vi "Main.vi"() -> ()   [LabVIEW 2021]
doc: "This template is for the Queued Message Handler design pattern.\n\nThe Event Handling Loop generates messages based on user interface actions.\n\nThe Message Handling Loop processes messages generated by the Event Handling Loop, or by other messages. The messages are string values, so new messages can be added easily to the Message Cases case structure in the Message Handling Loop. Each message cluster can also provide an optional value for Message Data, which is a variant that can be converted to whatever message-specific data is required."
uses:
  Controls/Status Lights.ctl
  controls/UI Data.ctl
  support/Message Queue/Enqueue Message (Single).vi
  <vilib>/Utility/error.llb/Error Cluster From Error Code.vi
  <vilib>/ErrorRing/Error Ring.xnode
  support/Message Queue/Message Queue.lvlib
  support/User Event - Stop/User Event - Stop.lvlib
panel:
  out "Status":T1
  in  "Speed":dbl(knob) scale=0.0..10.0
  out "Display":string
  in  "Direction":bool
  in  "Apply Brake":bool
  in  "Exit":bool
  # "These controls have associated \"Value Changed\" events configured in the Event Structure on the diagram.\n\nReplace them (and reconfigure the Event Structure) with the controls you need for your application."
  # "This template is for the Queued Message Handler design pattern.\n\nSee the block diagram for more information on how to use this template."
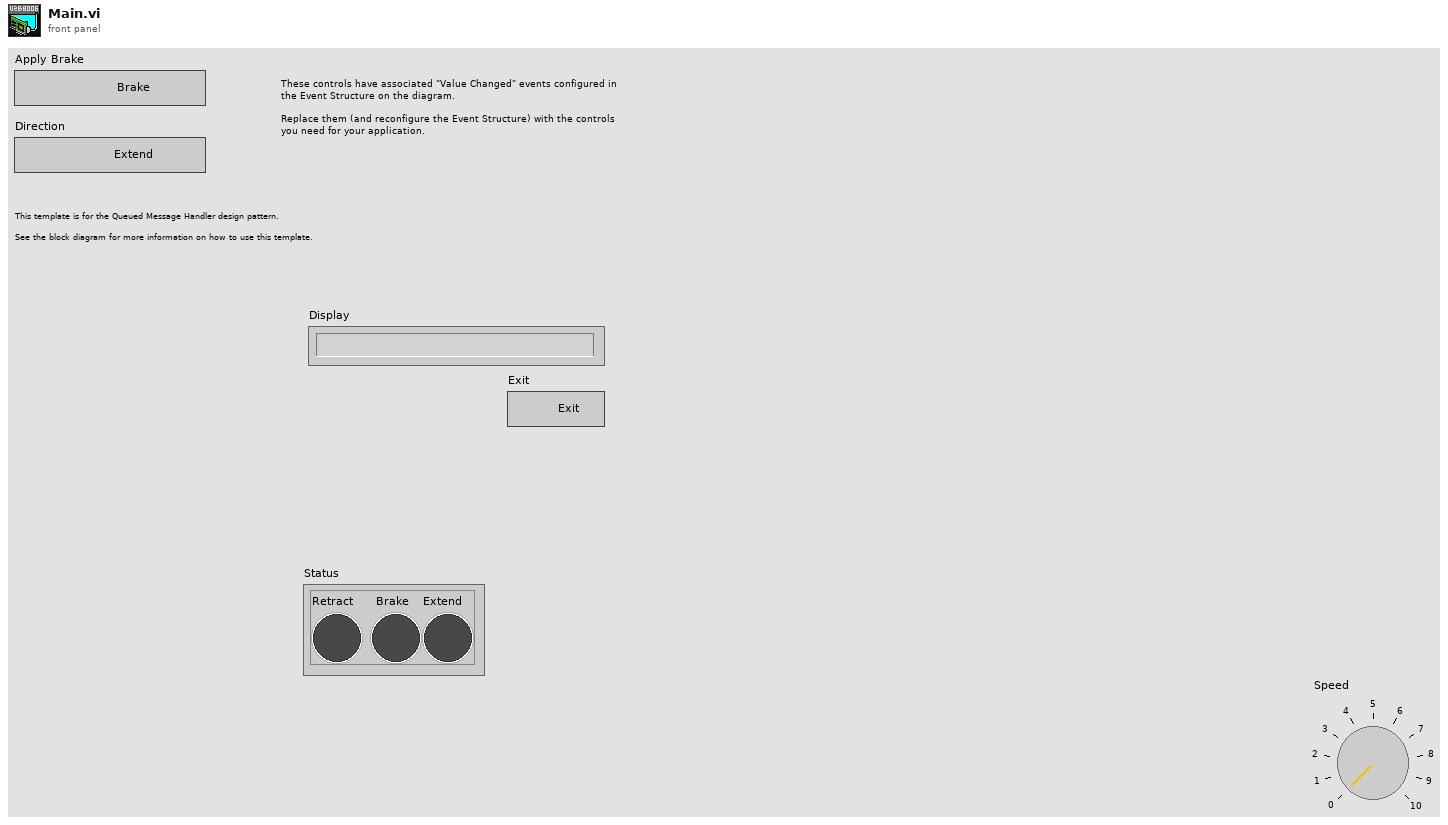
[diagram p1: front panel]
types:
  T1 = typedef "Status Lights.ctl" = cluster{"Retract":bool, "Brake":bool, "Extend":bool}
  T2 = typedef "UI Data.ctl" = cluster{"Boolean":bool, "String":string, "Velocity":dbl, "Apply Brake Ref":refnum<vi>, "Direction Ref":refnum<vi>, "Data Display Ref":refnum<vi>, "Exit Button Ref":refnum<vi>, "Status":T1}
  T3 = typedef "Message Queue.lvlib/All Message Queues.ctl" = cluster{"UI":refnum<queue>}
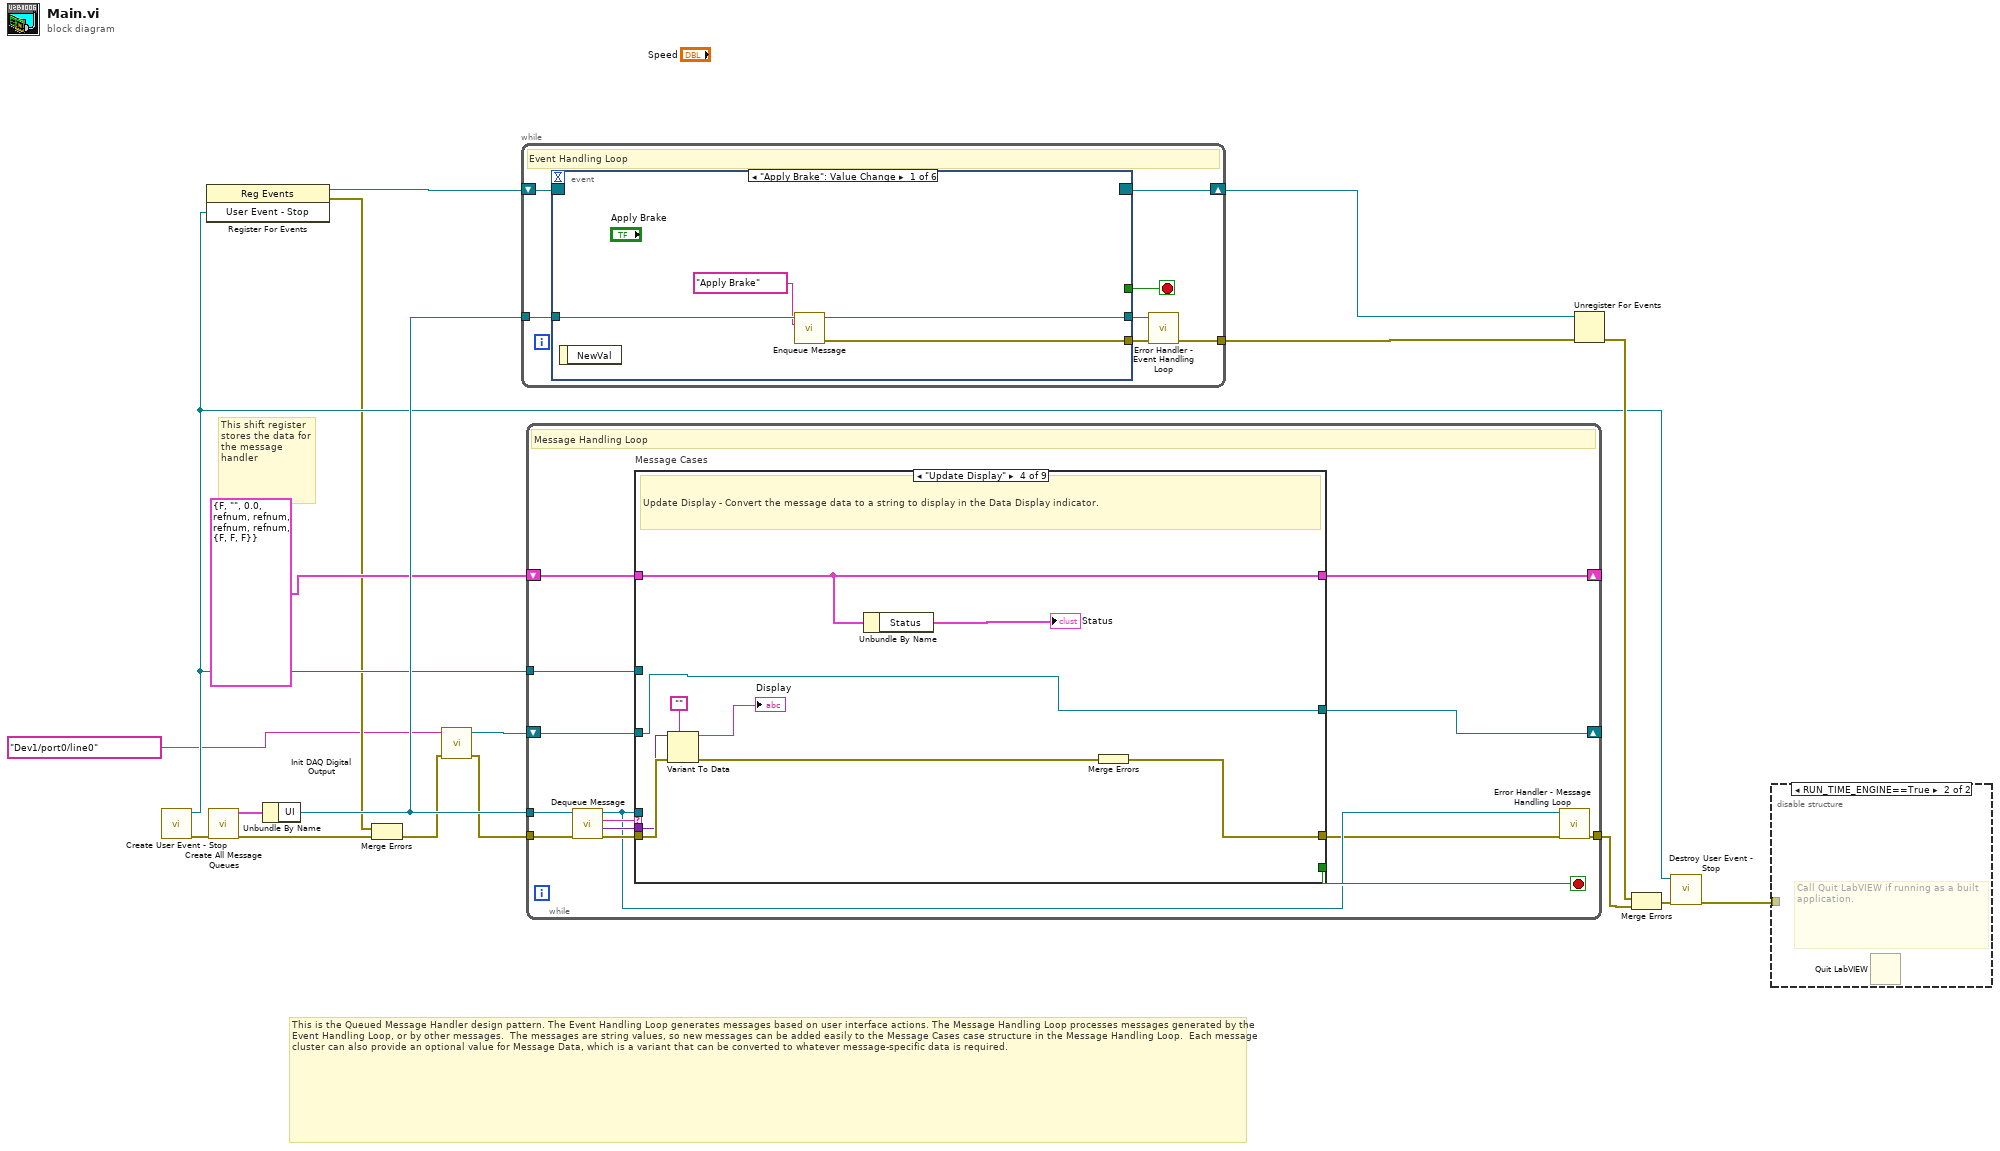
[diagram p0: block diagram]
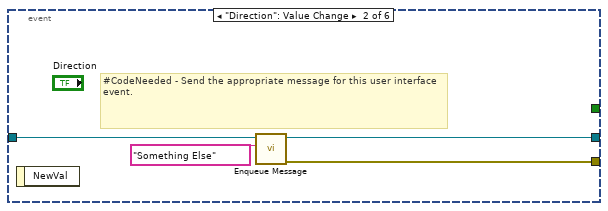
[diagram p3: hidden frame]
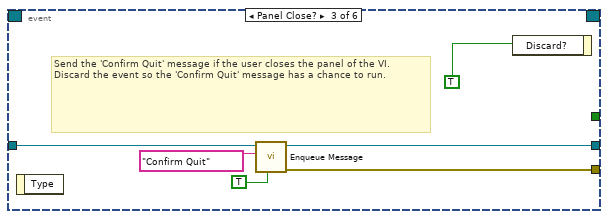
[diagram p4: hidden frame]
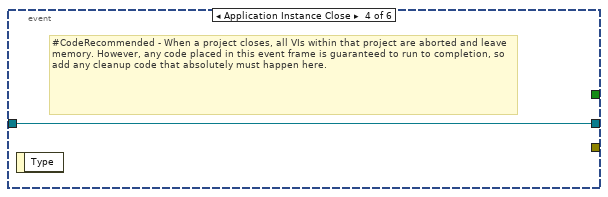
[diagram p5: hidden frame]
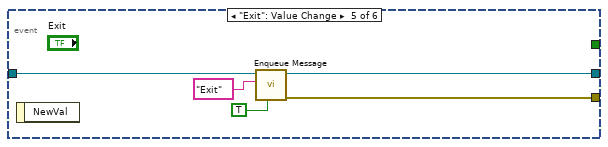
[diagram p6: hidden frame]
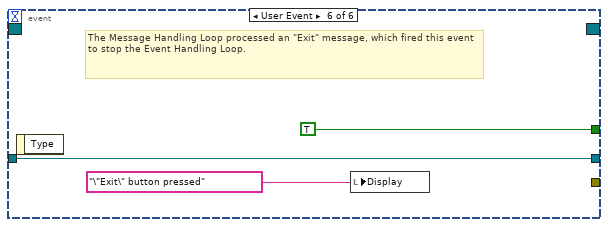
[diagram p7: hidden frame]
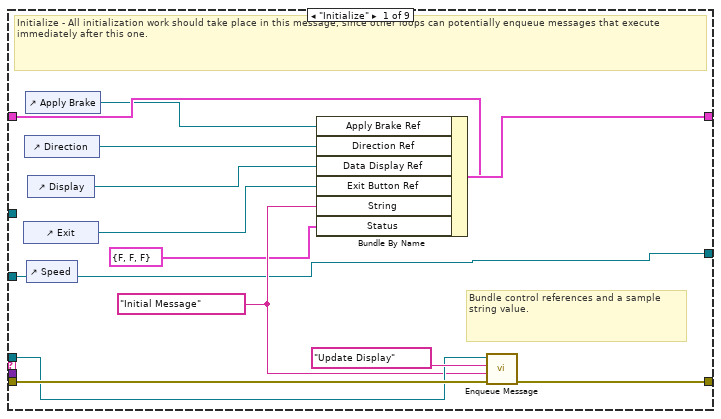
[diagram p8: hidden frame]
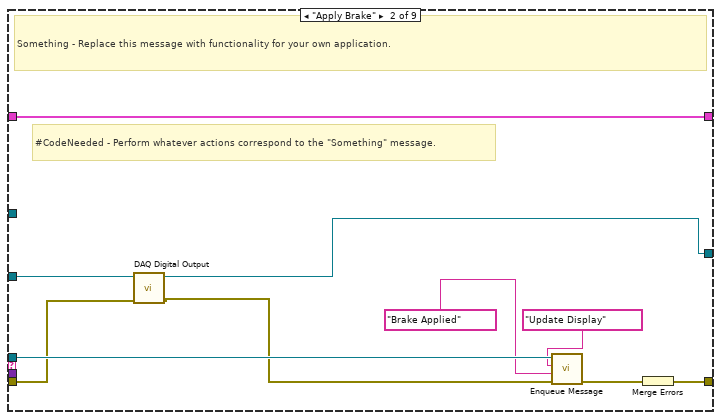
[diagram p9: hidden frame]
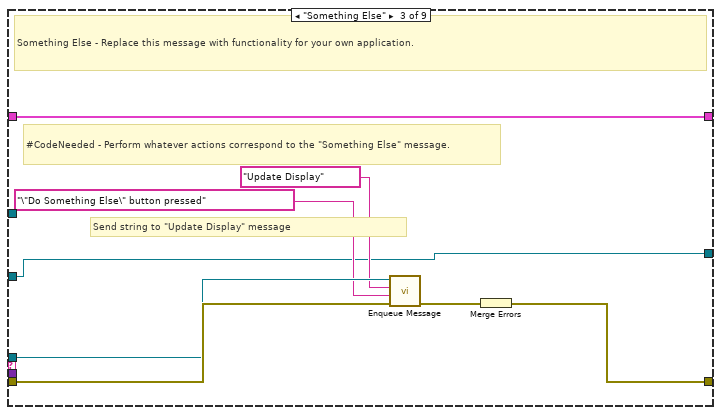
[diagram p10: hidden frame]
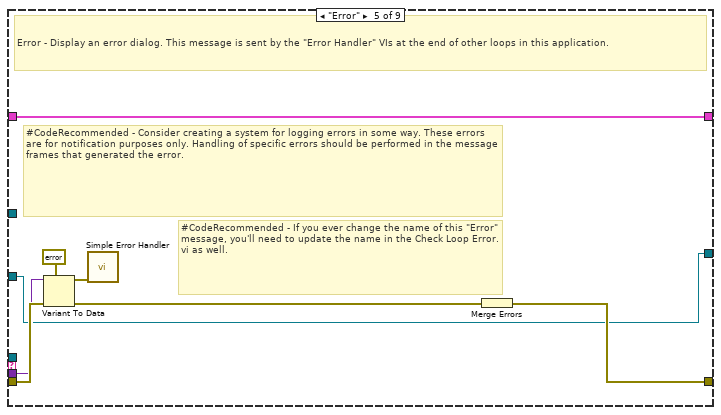
[diagram p11: hidden frame]
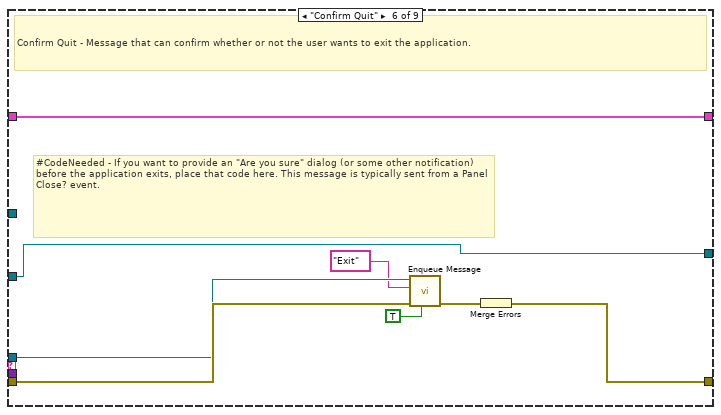
[diagram p12: hidden frame]
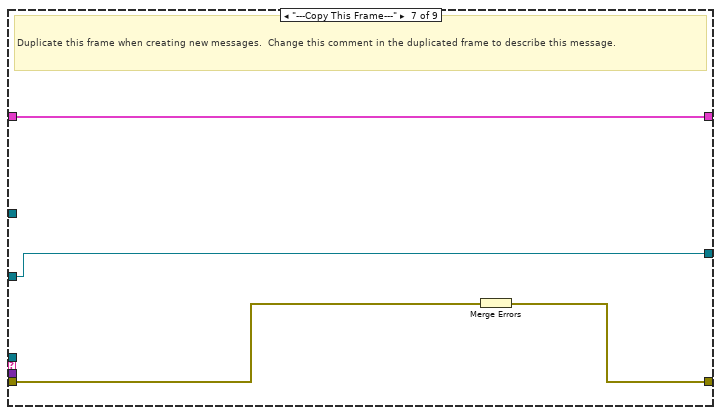
[diagram p13: hidden frame]
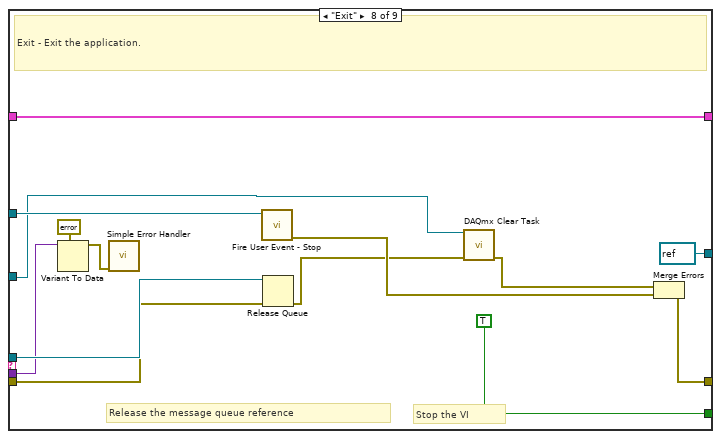
[diagram p14: hidden frame]
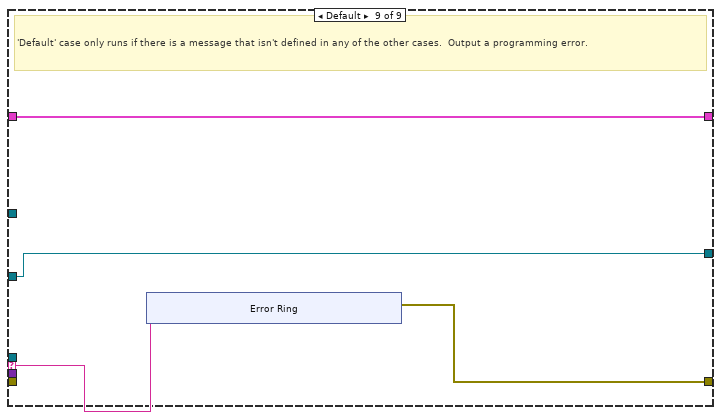
[diagram p15: hidden frame]
diagram:
  # "This is the Queued Message Handler design pattern. The Event Handling Loop generates messages based on user interface actions. The Message Handling Loop processes messages generated by the Event Handling Loop, or by other messages.  The messages are string values, so new messages can be added easily to the Message Cases case structure in the Message Handling Loop.  Each message cluster can also provide an optional value for Message Data, which is a variant that can be converted to whatever message-specific data is required."
  # "This shift register stores the data for the message handler"
  n1 = call "Create User Event - Stop.vi"() -> ("error out"=w15:errorcluster, "User Event - Stop"=w7:refnum<user-event>)  [unwired: 10 in]
  n2 = register-events(w7) -> (reference out=w8:refnum<event-registration>, error out=w6:errorcluster)  [unwired: 2 in]
  n3 = call "Create All Message Queues.vi"("error in (no error)"=w15) -> ("error out"=w18:errorcluster, "Message Queues out"=w17:T3)  [unwired: 9 in]
  n4 = Unbundle By Name(w17) -> ("UI"=w16:refnum<queue>)
  n5 = Merge Errors(w6, w18) -> (w4:errorcluster)
  n6 = call "Init DAQ Digital Output.vi"("error in"=w4, "lines"=tag "Dev1/port0/line0") -> ("error out"=w3:errorcluster, "Refnum out"=w5:refnum<k21>)  [unwired: 8 in]
  n7 = while {
    tunnel: w16 -> [w25]
    shift-right: [w23] -> w12
    shift-left: w8 -> [w24]
    tunnel: [w19] -> w9
    stop <- w21 stop-if-true
    # "Event Handling Loop"
    n8 = event shown="[0] \"Apply Brake\": Value Change" {
      selector: w24 -> [_ _ _ _ _ _]
      dyn-events: [_ _ _ _ _ _] -> w23
      timeout: _ -> [_ _ _ _ _ _]
      tunnel: [_ _ _ _ _ TRUE ("Discard?")] -> w21
      tunnel: w25 -> [w29 w33 w38 w40 w45 w48]
      tunnel: [w26 w30 w37 _ w44 _] -> w22
      tunnel: [w28 w32 w36 w40 w43 w48] -> w20
      event "Apply Brake": Value Change {
        n9 = event-data() -> ()  [unwired: 1 in, 1 out]
        n10 = call-poly "Enqueue Message.vi"("Message"="Apply Brake", "Message Queue"=w29) -> ("error out"=w26:errorcluster, "dup Message Queue"=w28:refnum<queue>)  [unwired: 8 in]
      }
      event "Direction": Value Change {
        # "#CodeNeeded - Send the appropriate message for this user interface event."
        n11 = event-data() -> ()  [unwired: 1 in, 1 out]
        n12 = call-poly "Enqueue Message.vi"("Message"="Something Else", "Message Queue"=w33) -> ("error out"=w30:errorcluster, "dup Message Queue"=w32:refnum<queue>)  [unwired: 8 in]
      }
      event Panel Close? {
        # "Send the 'Confirm Quit' message if the user closes the panel of the VI. Discard the event so the 'Confirm Quit' message has a chance to run."
        n13 = event-data() -> ()  [unwired: 1 in, 1 out]
        n14 = call-poly "Enqueue Message.vi"("Priority Message? (F)"=TRUE, "Message"="Confirm Quit", "Message Queue"=w38) -> ("error out"=w37:errorcluster, "dup Message Queue"=w36:refnum<queue>)  [unwired: 7 in]
        n15 = event-data("Discard?"=TRUE) -> ()  [unwired: 1 in, 1 out]
      }
      event Application Instance Close {
        # "#CodeRecommended - When a project closes, all VIs within that project are aborted and leave memory. However, any code placed in this event frame is guaranteed to run to completion, so add any cleanup code that absolutely must happen here."
        n16 = event-data() -> ()  [unwired: 1 in, 1 out]
      }
      event "Exit": Value Change {
        n17 = event-data() -> ()  [unwired: 1 in, 1 out]
        n18 = call-poly "Enqueue Message.vi"("Priority Message? (F)"=TRUE, "Message"="Exit", "Message Queue"=w45) -> ("error out"=w44:errorcluster, "dup Message Queue"=w43:refnum<queue>)  [unwired: 7 in]
      }
      event User Event {
        # "The Message Handling Loop processed an \"Exit\" message, which fired this event to stop the Event Handling Loop."
        n19 = event-data() -> ()  [unwired: 1 in, 1 out]
        n20 = local write "Display"("\"Exit\" button pressed" ("VI Stopped")) -> ()
      }
    }
    n21 = call "Error Handler - Event Handling Loop.vi"("error in (no error)"=w22, "Message Queue"=w20) -> ("dup error in"=w19:errorcluster)  [unwired: 8 in, 1 out]
  }
  n22 = while {
    tunnel: w16 -> [w54]
    shift-right: [w61] -> _
    shift-left: T2 {"Boolean"=FALSE, "String"="", "Velocity"=0.0, "Apply Brake Ref"=refnum, "Direction Ref"=refnum, "Data Display Ref"=refnum, "Exit Button Ref"=refnum, "Status"={"Retract"=FALSE, "Brake"=FALSE, "Extend"=FALSE}} ("Data Cluster") -> [w62]
    tunnel: w7 -> [w59]
    tunnel: w3 -> [w58]
    tunnel: [w52] -> w1
    shift-right: [w50] -> _
    shift-left: w5 -> [w49]
    stop <- w60 stop-if-true
    # "Message Handling Loop"
    n23 = call "Dequeue Message.vi"("error in (no error)"=w58, "Message Queue"=w54) -> ("error out"=w57:errorcluster, "Message Data"=w55:variant, "Message"=w56:string, "dup Message Queue"=w53:refnum<queue>)  [unwired: 6 in]
    n24 = case "Message Cases" shown="\"Update Display\"" w56 {
      selector: w56 -> [_ _ _ _ _ _ _ _ w138]
      tunnel: w53 -> [w68 w82 w89 _ _ w114 _ w136 _]
      tunnel: w57 -> [w74 w78 w91 w101 w110 w118 w122 w130 _]
      tunnel: [w75 w84 w92 w102 w104 w116 w120 w133 w139] -> w51
      tunnel: w62 -> [w66 w85 w93 w95 w109 w117 w121 w135 w140]
      tunnel: [w73 w85 w93 w95 w109 w117 w121 w135 w140] -> w61
      tunnel: [_ _ _ _ _ _ _ TRUE _] -> w60
      tunnel: w55 -> [_ _ _ w100 w108 _ _ w127 _]
      tunnel: w59 -> [_ _ _ _ _ _ _ w132 _]
      tunnel: [w65 w76 w86 w96 w103 w111 w119 refnum<k21> refnum ("Refnum out") w137] -> w50
      tunnel: w49 -> [w65 w79 w86 w96 w103 w111 w119 w126 w137]
      frame "Initialize" {
        w67 = "Initial Message" ("Initial Message")
        # "Bundle control references and a sample string value."
        # "Initialize - All initialization work should take place in this message, since other loops can potentially enqueue messages that execute immediately after this one."
        n25 = control-ref of="Exit"() -> (w70:refnum<vi>)
        n26 = control-ref of="Direction"() -> (w72:refnum<vi>)
        n27 = control-ref of="Apply Brake"() -> (w64:refnum<vi>)
        n28 = control-ref of="Speed"() -> ()  [unwired: 1 out]
        n29 = control-ref of="Display"() -> (w71:refnum<vi>)
        n30 = Bundle By Name(cluster=w66, "Apply Brake Ref"=w64, "Direction Ref"=w72, "Data Display Ref"=w71, "Exit Button Ref"=w70, "String"=w67, "Status"=T1 {"Retract"=FALSE, "Brake"=FALSE, "Extend"=FALSE}) -> (w73:T2)
        n31 = call-poly "Enqueue Message.vi"("error in (no error)"=w74, "Message Data"=w67, "Message"="Update Display", "Message Queue"=w68) -> ("error out"=w75:errorcluster)  [unwired: 6 in, 1 out]
      }
      frame "Apply Brake" {
        # "#CodeNeeded - Perform whatever actions correspond to the \"Something\" message."
        # "Something - Replace this message with functionality for your own application."
        n32 = call "DAQ Digital Output.vi"("error in"=w78, "task/channels in"=w79) -> ("error out"=w77:errorcluster, "task out"=w76:refnum<k21>)  [unwired: 7 in, 1 out]
        n33 = call-poly "Enqueue Message.vi"("error in (no error)"=w77, "Message Data"="Brake Applied" ("\"Do Something\" button pressed"), "Message"="Update Display", "Message Queue"=w82) -> ("error out"=w83:errorcluster)  [unwired: 6 in, 1 out]
        n34 = Merge Errors(w83) -> (w84:errorcluster)
      }
      frame "Something Else" {
        # "Send string to \"Update Display\" message"
        # "#CodeNeeded - Perform whatever actions correspond to the \"Something Else\" message."
        # "Something Else - Replace this message with functionality for your own application."
        n35 = call-poly "Enqueue Message.vi"("error in (no error)"=w91, "Message Data"="\"Do Something Else\" button pressed" ("\"Do Something Else\" button pressed"), "Message"="Update Display", "Message Queue"=w89) -> ("error out"=w90:errorcluster)  [unwired: 6 in, 1 out]
        n36 = Merge Errors(w90) -> (w92:errorcluster)
      }
      frame "Update Display" {
        # "Update Display - Convert the message data to a string to display in the Data Display indicator."
        n37 = Variant To Data(error in=w101, type="", Variant=w100) -> (data=→"Display":string, error out=w98:errorcluster)
        n38 = Unbundle By Name(w95) -> ("Status"=→"Status":T1)
        n39 = Merge Errors(w98) -> (w102:errorcluster)
      }
      frame "Error" {
        # "#CodeRecommended - If you ever change the name of this \"Error\" message, you'll need to update the name in the Check Loop Error.vi as well."
        # "#CodeRecommended - Consider creating a system for logging errors in some way. These errors are for notification purposes only. Handling of specific errors should be performed in the message frames that generated the error."
        # "Error - Display an error dialog. This message is sent by the \"Error Handler\" VIs at the end of other loops in this application."
        n40 = Variant To Data(error in=w110, type=errorcluster {"status"=FALSE, "code"=0, "source"=""} ("error constant"), Variant=w108) -> (data=w106:errorcluster, error out=w105:errorcluster)
        n41 = call <vilib>:"Simple Error Handler.vi"("error in (no error)"=w106) -> ()  [unwired: 4 in, 5 out]
        n42 = Merge Errors(w105) -> (w104:errorcluster)
      }
      frame "Confirm Quit" {
        # "#CodeNeeded - If you want to provide an \"Are you sure\" dialog (or some other notification) before the application exits, place that code here. This message is typically sent from a Panel Close? event."
        # "Confirm Quit - Message that can confirm whether or not the user wants to exit the application."
        n43 = call-poly "Enqueue Message.vi"("Priority Message? (F)"=TRUE, "error in (no error)"=w118, "Message"="Exit", "Message Queue"=w114) -> ("error out"=w115:errorcluster)  [unwired: 6 in, 1 out]
        n44 = Merge Errors(w115) -> (w116:errorcluster)
      }
      frame "---Copy This Frame---" {
        # "Duplicate this frame when creating new messages.  Change this comment in the duplicated frame to describe this message."
        n45 = Merge Errors(w122) -> (w120:errorcluster)
      }
      frame "Exit" {
        # "Stop the VI"
        # "Release the message queue reference"
        # "Exit - Exit the application."
        n46 = Variant To Data(type=errorcluster {"status"=FALSE, "code"=0, "source"=""} ("error constant"), Variant=w127) -> (data=w128:errorcluster)  [unwired: 1 in, 1 out]
        n47 = call <vilib>:"Simple Error Handler.vi"("error in (no error)"=w128) -> ()  [unwired: 4 in, 5 out]
        n48 = call "Fire User Event - Stop.vi"("User Event - Stop"=w132) -> ("error out"=w131:errorcluster)  [unwired: 10 in]
        n49 = Release Queue(queue=w136, error in (no error)=w130) -> (error out=w124:errorcluster)  [unwired: 1 in, 2 out]
        n50 = call <vilib>:"DAQmx Clear Task.vi"("task in"=w126, "error in"=w124) -> ("error out"=w125:errorcluster)  [unwired: 13 in]
        n51 = Merge Errors(w125, w131) -> (w133:errorcluster)
      }
      frame Default {
        # "'Default' case only runs if there is a message that isn't defined in any of the other cases.  Output a programming error."
        n52 = xnode "Error Ring"("parameter 0"=w138) -> ("error out"=w139:errorcluster)
      }
    }
    n53 = call "Error Handler - Message Handling Loop.vi"("error in (no error)"=w51, "Message Queue"=w53) -> ("dup error in"=w52:errorcluster)  [unwired: 8 in, 1 out]
  }
  n54 = Unregister For Events(event registration refnum=w12, error in=w9) -> (error out=w13:errorcluster)
  n55 = Merge Errors(w13, w1) -> (w14:errorcluster)
  n56 = call "Destroy User Event - Stop.vi"("error in (no error)"=w14, "User Event - Stop"=w7) -> ("error out"=w10:errorcluster)  [unwired: 9 in]
  n57 = disable-structure shown="RUN_TIME_ENGINE==True" {
    disable-tunnel: w10 -> [_ _]
    frame condition #0 (active) {
    }
    frame condition #1 {
      # "Call Quit LabVIEW if running as a built application."
      n58 = Quit LabVIEW() -> ()  [unwired: 1 in]
    }
  }
